vi "FxLine.vi"(7 "采样频率":dbl=200.0, 8 "终点值":dbl, 9 "起点值":dbl, 10 "终点时间":dbl, 11 "起点时间":dbl) -> (0 "Y":dbl[](array[numeric]), 3 "X":dbl[](array[numeric]))   [LabVIEW 2020, in "Curve Editor.lvlib"]
uses:
  Curve Editor.lvlib
panel:
  out "XY图":cluster{dbl[], dbl[]}(graph)
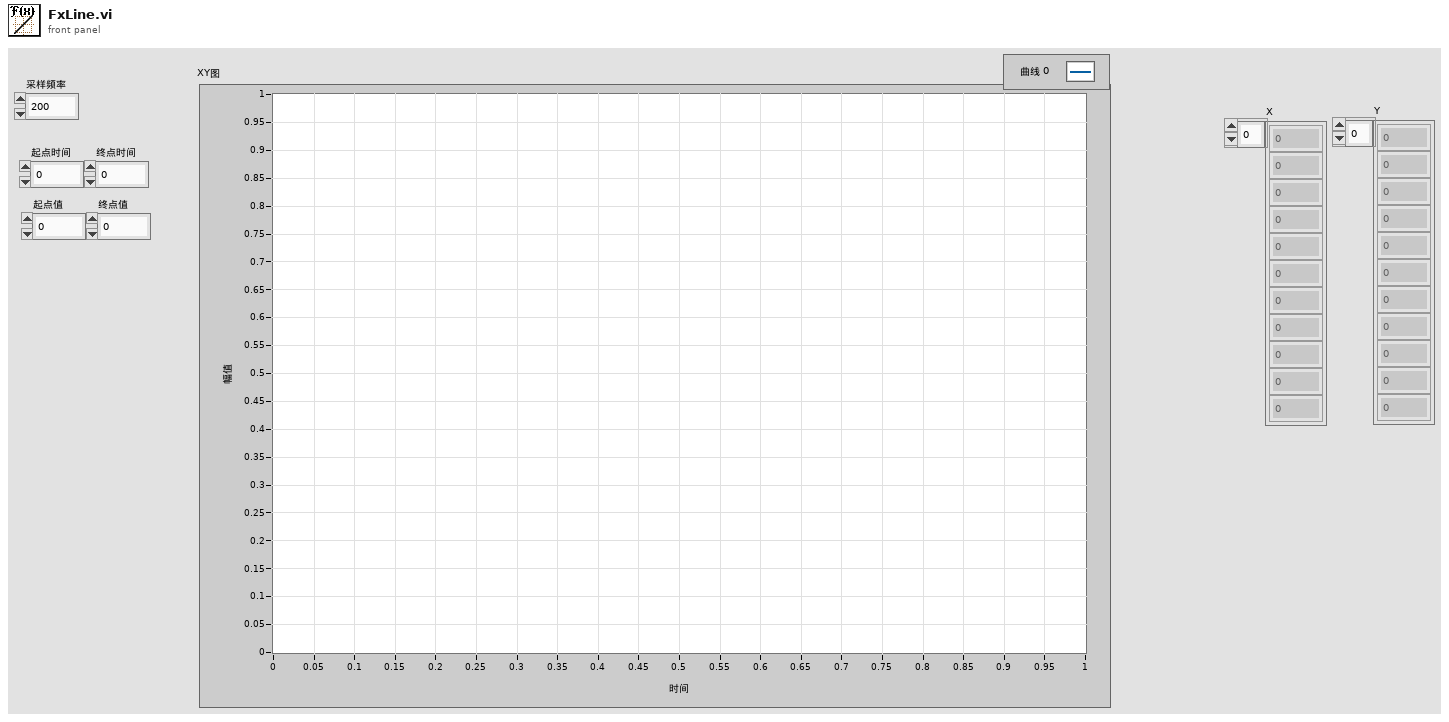
[diagram p1: front panel]
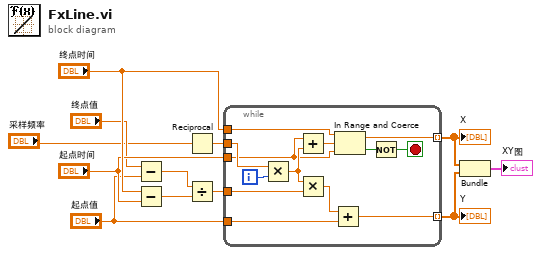
[diagram p0: block diagram]
diagram:
  n1 = Subtract(x="终点值", y="起点值") -> (x-y=w6:dbl)
  n2 = Subtract(x="终点时间", y="起点时间") -> (x-y=w5:dbl)
  n3 = Reciprocal(x="采样频率") -> (1/x=w11:dbl)
  n4 = Divide(x=w6, y=w5) -> (x/y=w3:dbl)
  n5 = while {
    tunnel: [w21] -> w12 mode=indexing
    tunnel: "起点时间" -> [w13]
    tunnel: "终点时间" -> [w25]
    tunnel: w11 -> [w23]
    tunnel: "起点值" -> [w18]
    tunnel: w3 -> [w16]
    tunnel: [w14] -> w2 mode=indexing
    i -> [w24]
    stop <- w19 stop-if-true
    n6 = Multiply(x=w23, y=w24) -> (x*y=w17:dbl)
    n7 = Add(x=w13, y=w17) -> (x+y=w22:dbl)
    n8 = Multiply(x=w17, y=w16) -> (x*y=w15:dbl)
    n9 = Add(x=w15, y=w18) -> (x+y=w14:dbl)
    n10 = In Range and Coerce(upper limit=w25, x=w22, lower limit=w13) -> (coerced(x)=w21:dbl, In Range?=w20:bool)
    n11 = Not(x=w20) -> (.not. x?=w19:bool)
  }
  "X" <- w12
  "Y" <- w2
  n12 = Bundle(w12, w2) -> (→"XY图":cluster{dbl[], dbl[]})  [unwired: 1 in]
